vi "practiceImageAnalysis - HH.vi"() -> ()   [LabVIEW 2016]
uses:
  <vilib>/vision/Image Controls.llb/IMAQ Image.ctl
  <vilib>/vision/Measure.llb/Edge Options.ctl
  <vilib>/vision/Measure.llb/Edge Polarity.ctl
  <vilib>/vision/NI_Vision_Development_Module.lvlib
  <vilib>/Analysis/NI_AALPro.lvlib
  <vilib>/Utility/file.llb/Write Delimited Spreadsheet (DBL).vi
panel:
  out "Fitted edge residue":dbl
  out "Fitted edge error":i32
  out "Fitted edge intercept":dbl
  out "Fitted edge slope":dbl
  in  "Linear fit parameter bounds":T1={"slope min"=-inf, "slope max"=inf, "intercept min"=-inf, "intercept max"=inf}
  out "x^2 fit error":i32
  out "Polynomial Coefficients":dbl[](array[numeric])
  out "Residuals":dbl[](array[numeric])
  out "Fitted SD( dI/dR )":dbl[](array[numeric])
  out "Fitted edge locations":dbl[](array[numeric])
  out "residue":dbl
  out "Fit residue vs Z":T2(graph)
  out "Fitted SD dI/dR vs Z":T3(graph)
  out "Fitted radii vs Z":T3(graph)
  out "Processing Image #":i32
  out "Derivative: Normalized Intensity vs Radius":T3(graph)
  out "Selected subarray":T4(plugin-control)
  out "Normalized Intensity vs Radius":cluster{dbl[], dbl[]}(graph)
  in  "nBins":dbl=300.0
  in  "Min":dbl
  in  "Max":dbl=300.0
  out "Fitted Circle":T5 {"Average SNR (dB)" format="%.2f"; "Average Strength" format="%.2f"; "Roundness (Real-World)" format="%.2f"; "Radius (Real-World)" format="%.2f"; "Center (Real-World)"."Y" format="%.2f"; "Center (Real-World)"."X" format="%.2f"; "Radius (Pixels)" format="%.2f"; "Center (Pixels)"."Y" format="%.2f"; "Center (Pixels)"."X" format="%.2f"}
  out "Npixel@Intensity Histogram":T6(graph)
  out "Npixel@phi Histogram":T6(graph)
  out "Npixel@R Histogram":T6(graph)
  in  "Circle ROI Descriptor":T7={"Global Rectangle"=[675, 567, 1751, 1642], "Contours"=[{"ID"=enum."External", "Type"=7, "Coordinates"=[1212, 1104, 85, 537, 0, 0]}]} {"Contours"."Type" items=["No Selection", "Point", "Line", "Rectangle", "Oval", "Polygon", "Freehand Region", "Annulus", "Unused2", "Unused3", "Broken Line", "Freehand Line", "Rotated Rectangle"]}
  in  "Circle Fit Options":T8={"Process"=enum."Get Best Edge", "Step Size"=3.0, "Max Pixel Radius"=3}
  in  "Circle Finding Options":T11={"Search  Direction"=1, "Edge Options"={"Edge Polarity"=2, "Kernel Size"=3, "Width"=3, "Minimum Edge Strength"=10.0, "Interpolation Type"=enum."Bilinear Fixed", "Data Processing Method"=enum."Average"}, "Show Search Area"=FALSE, "Show Search Lines"=FALSE, "Show Edges Found"=FALSE, "Show Result"=TRUE, "Search Area Color"=65280, "Search Lines Color"=255, "Edge Locations Color"=16776960, "Result Color"=65511, "Overlay Group Name"=""} {"Search  Direction" items=["Outside to Inside", "Inside to Outside"]; "Edge Options"."Edge Polarity" items=["All Edges", "Rising Edges", "Falling Edges"]; "Edge Options"."Minimum Edge Strength" format="%.2f"; "Edge Options"."Width" step=2; "Edge Options"."Kernel Size" step=2}
  in  "Pattern Match Settings":T12={"Algorithm"=2, "Number of Matches Requested"=1, "Minimum Match Score"=800.0, "SubPixel Accuracy"=TRUE, "Rotation Angle Ranges"=[], "Show Search Area"=FALSE, "Show Result"=TRUE} {"Rotation Angle Ranges"."End" format="%.1f"; "Rotation Angle Ranges"."Start" format="%.1f"; "Minimum Match Score" min=0 max=1000 format="%.2f"; "Number of Matches Requested" min=1; "Algorithm" items=["All", "Low Discrepancy Sampling", "Grayscale Value Pyramid", "Gradients Pyramid"]}
  out "Template Image":T4
  in  "Coordinate file for image capture":path=path "C:/Users/sciollalab/Desktop/dotCoordinates-captured.csv"
  out "Review":bool
  out "Search running?":bool
  in  "Stop and delete":bool
  out "Images Array":T4[](array[plugin-control])=["image_442_-22_00"]
  in  "error in":errorcluster
  out "error out":errorcluster
  out "Filenames Array":string[](array[string])
  in  "Naming Convention":string="image_442_-22_00.png"
  in  "Images Directory":path=path "C:/Users/sciollalab/Desktop/dots1-12-16-2016/dots_-146,-22"
  # "add linear fit to R vs Z"
  # "fit to a parabola"
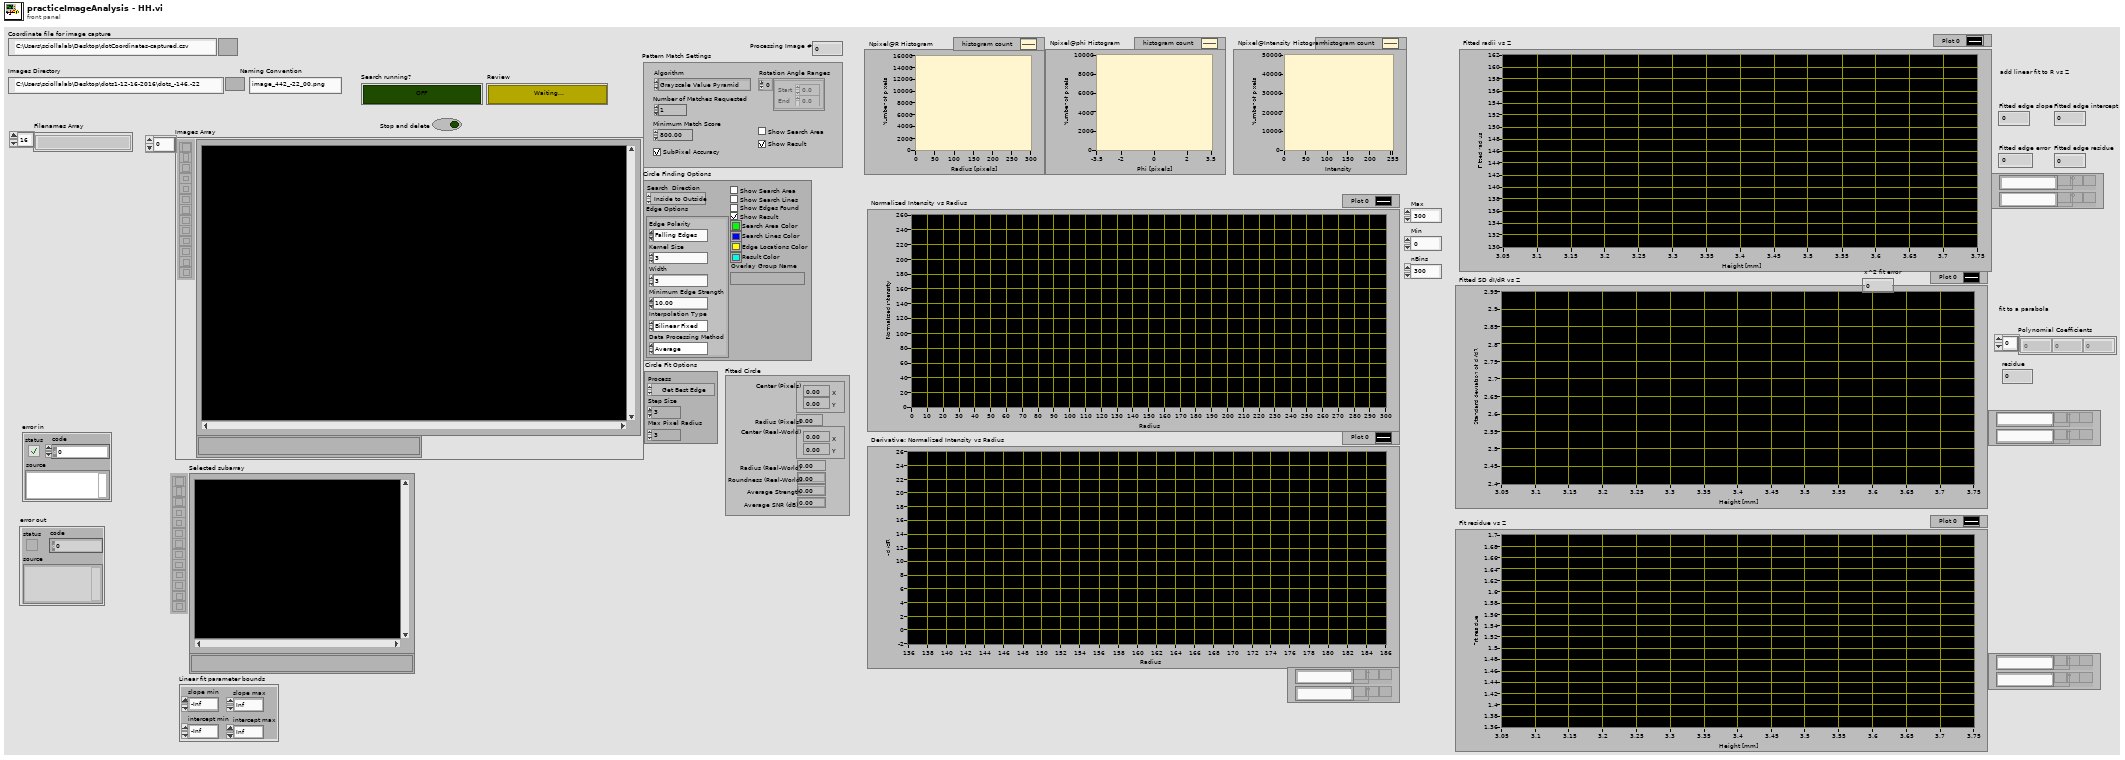
[diagram p1: front panel]
types:
  T1 = cluster{"slope min":dbl, "slope max":dbl, "intercept min":dbl, "intercept max":dbl}
  T2 = cluster{"Image coordinates in lab frame":dbl[], dbl[]}
  T3 = cluster{"Radius bins":dbl[], "Best Gaussian Fit":dbl[]}[]
  T4 = typedef "IMAQ Image.ctl" = refnum<image>
  T5 = cluster{"Center (Pixels)":cluster{"X":sgl, "Y":sgl}, "Radius (Pixels)":dbl, "Center (Real-World)":cluster{"X":sgl, "Y":sgl}, "Radius (Real-World)":dbl, "Roundness (Real-World)":dbl, "Average Strength":dbl, "Average SNR (dB)":dbl}
  T6 = cluster{"X Values":dbl[], "Histogram: h(x)":i32[]}
  T7 = cluster{"Global Rectangle":i32[], "Contours":cluster{"ID":enum32{"External", "Internal"}, "Type":u32, "Coordinates":i32[]}[]}
  T8 = cluster{"Process":enum16{"Get First Edge", "Get First + Last Edge", "Get All Edges", "Get Best Edge"}, "Step Size":dbl, "Max Pixel Radius":i32}
  T9 = typedef "Edge Options.ctl" = cluster{"Edge Polarity":T10, "Kernel Size":u32, "Width":u32, "Minimum Edge Strength":sgl, "Interpolation Type":enum32{"Zero Order", "Bilinear", "Quadratic", "Cubic", "Bilinear Fixed"}, "Data Processing Method":enum32{"Average", "Median"}}
  T10 = typedef "Edge Polarity.ctl" = u32
  T11 = cluster{"Search  Direction":u32, "Edge Options":T9, "Show Search Area":bool, "Show Search Lines":bool, "Show Edges Found":bool, "Show Result":bool, "Search Area Color":u32, "Search Lines Color":u32, "Edge Locations Color":u32, "Result Color":u32, "Overlay Group Name":string}
  T12 = cluster{"Algorithm":i32, "Number of Matches Requested":i32, "Minimum Match Score":sgl, "SubPixel Accuracy":bool, "Rotation Angle Ranges":cluster{"Start":sgl, "End":sgl}[], "Show Search Area":bool, "Show Result":bool}
  T13 = enum16{"cm", "mm", "pixels [mm/pix]", "pixels [um/pix]"}
  T14 = cluster{"Position":cluster{"x":sgl, "y":sgl}, "Angle":sgl, "Scale":sgl, "Score":sgl, "Bounding Box":cluster{"x":sgl, "y":sgl}[]}[]
  T15 = cluster{"Global Rectangle":i32[], cluster{"ID":enum32{"External", "Internal"}, "Type":u32, "Coordinates":i32[]}[]}
  T16 = cluster{"initial amplitude":dbl, "initial center":dbl, "initial standard deviation":dbl, "offset":dbl}
  T17 = cluster{"Image coordinates in lab frame":dbl[], "Residuals":dbl[]}
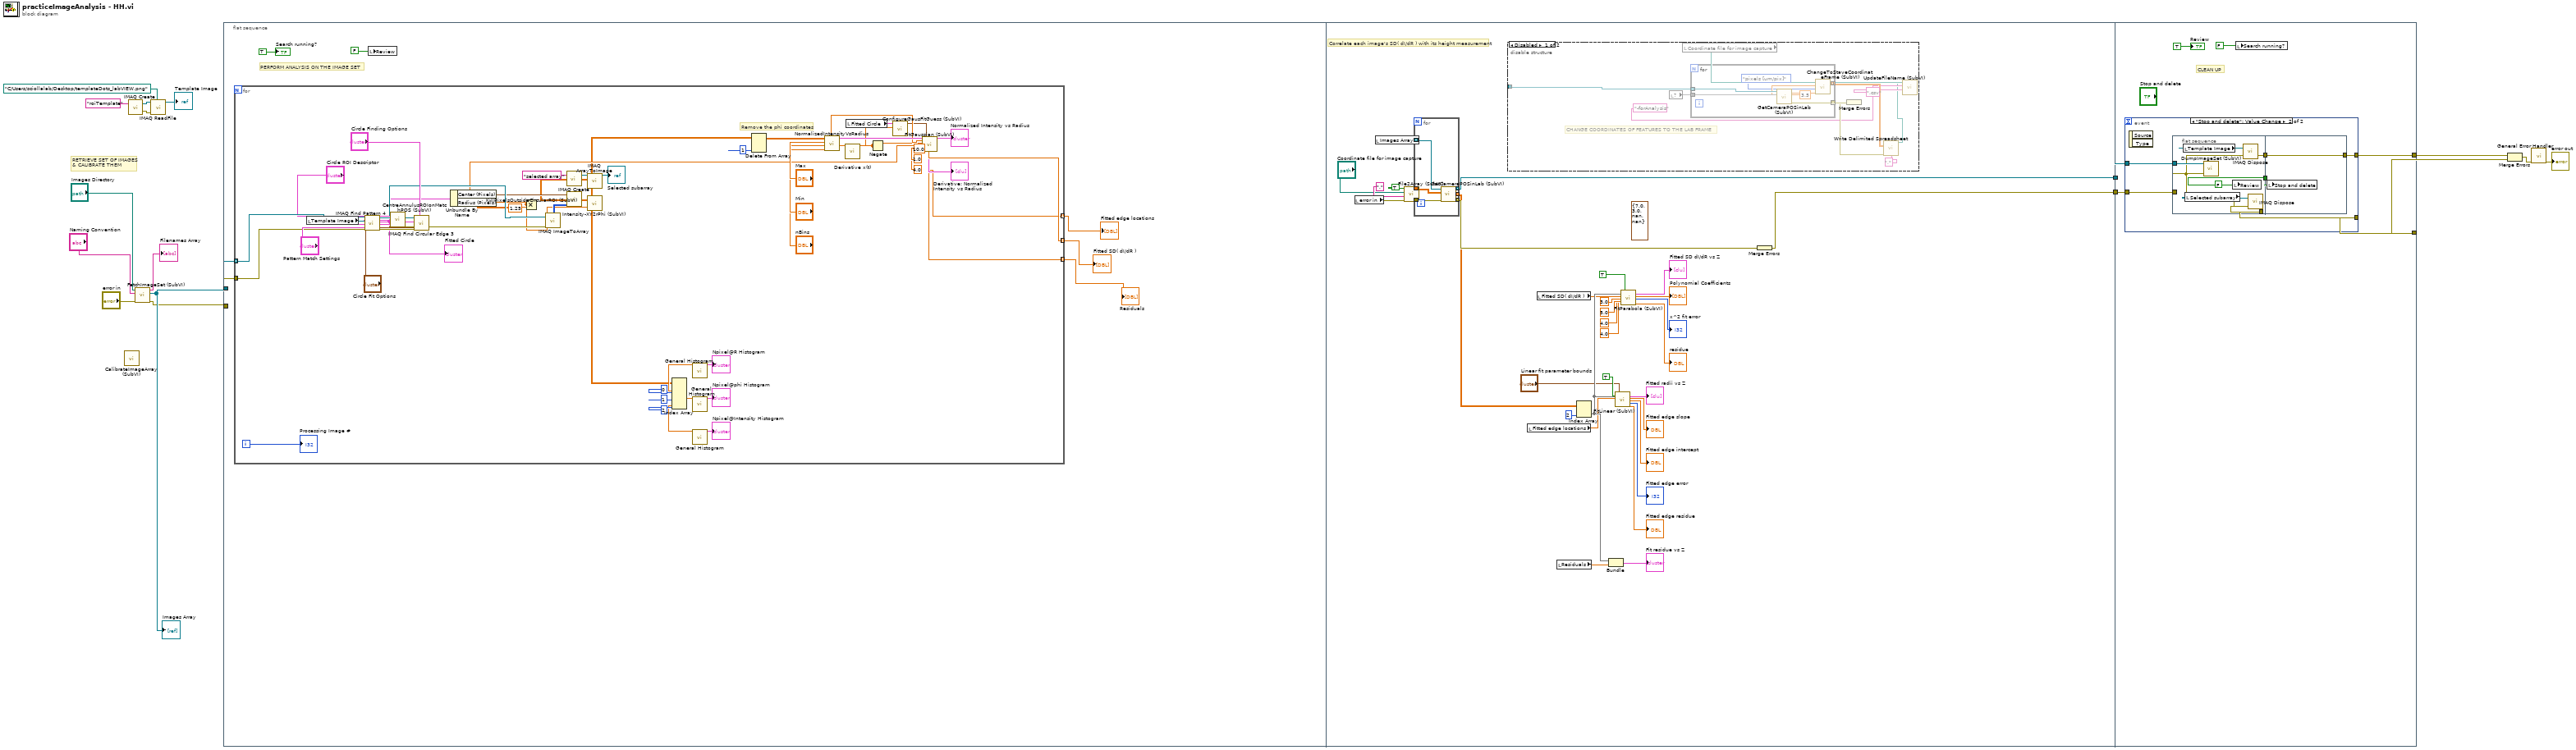
[diagram p0: block diagram]
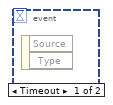
[diagram p3: hidden frame]
diagram:
  # "RETRIEVE SET OF IMAGES\n& CALIBRATE THEM"
  n1 = call "CalibrateImageArray (SubVI).vi"() -> ()  [unwired: 9 in, 2 out]
  n2 = call "IMAQ Create"("Image Name"="roiTemplate") -> ("New Image"=w7:T4, "error out"=w8:errorcluster)  [unwired: 4 in]
  n3 = call "FetchImageSet (SubVI).vi"("error in (no error)"="error in", "Naming Convention"="Naming Convention", "Images Directory"="Images Directory") -> ("error out"=w4:errorcluster, "Image Array"=w10:T4[], "Filenames Array"=→"Filenames Array":string[])  [unwired: 6 in]
  "Images Array" <- w10
  n4 = call "IMAQ ReadFile"("File Path"=path "C:/Users/sciollalab/Desktop/templateDots_labVIEW.png" ("Template File Path"), "error in (no error)"=w8, "Image"=w7) -> ("Image Out"=→"Template Image":T4)  [unwired: 4 in, 4 out]
  n5 = flat-sequence {
    tunnel: w10 -> [w22]
    tunnel: w4 -> [w21]
    tunnel: [w104] -> w3
    tunnel: [w102] -> w2
    tunnel: [w138] -> w12
    tunnel: w3 -> [w137]
    tunnel: w2 -> [w136]
    tunnel: [w135] -> w1
    frame #0 {
      # "PERFORM ANALYSIS ON THE IMAGE SET"
      n6 = for {
        tunnel: w22 -> [w77] mode=indexing
        tunnel: w21 -> [w75]
        tunnel: [w36] -> w19 mode=indexing
        tunnel: [w34] -> w18 mode=indexing
        tunnel: [w33] -> w20 mode=indexing
        i -> [w37]
        # "Remove the phi coordinates"
        n7 = local read "Template Image"() -> (w78:T4)
        n8 = call "IMAQ Find Pattern 4"("Image"=w77, "Template"=w78, "error in"=w75, "Settings"="Pattern Match Settings") -> ("Image Out"=w69:T4, "Matches (pixel)"=w71:T14, "error out"=w68:errorcluster)  [unwired: 5 in, 4 out]
        n9 = call "CentreAnnulusROIonMatchPOS (SubVI).vi"("Matches (pixel)"=w71, "Annulus ROI Descriptor"="Circle ROI Descriptor") -> ("Annulus ROI Descriptor centred on match position"=w70:T15)
        n10 = call "IMAQ Find Circular Edge 3"("Circle Fit Options"="Circle Fit Options", "Options"="Circle Finding Options", "error in (no error)"=w68, "ROI Descriptor"=w70, "Image"=w69) -> ("error out"=w67:errorcluster, "Fitted Circle"=w30:T5, "Image Out"=w59:T4)  [unwired: 2 in, 2 out]
        "Fitted Circle" <- w30
        n11 = Unbundle By Name(w30) -> ("Center (Pixels)"=w56:cluster{"X":sgl, "Y":sgl}, "Radius (Pixels)"=w38:dbl)
        n12 = Multiply(x=w38, y=1.25) -> (x*y=w44:dbl)
        n13 = call "IMAQ ImageToArray"("error in (no error)"=w67, "Image"=w59) -> ("Image Pixels (U8)"=w57:u8[][])  [unwired: 2 in, 4 out]
        n14 = call "IMAQ Create"("Image Name"="selected array") -> ("New Image"=w47:T4)  [unwired: 4 in, 1 out]
        n15 = call "KillPixelsOutsideCircularROI (SubVI).vi"("XY Array"=w57, "Radius*ScaleFactor"=w44, "Center (Pixels)"=w56) -> ("subarray"=w46:dbl[][])
        n16 = call "IMAQ ArrayToImage"("Image Pixels (U8)"=w46, "Image"=w47) -> ("Image Out"=→"Selected subarray":T4)  [unwired: 8 in, 1 out]
        n17 = call "Intensity-XY2rPhi (SubVI).vi"("Radius*Scale Factor"=w44, "XY Array"=w46) -> ("2D Array: r, phi, intensity"=w32:dbl[][])  [unwired: 1 out]
        n18 = Index Array(array=w32, index (col) #1=0 ("disabled index (col)"), index (col) #2=1 ("index (col)"), index (col) #3=2 ("index (col)")) -> (element #1=w55:dbl[], element #2=w60:dbl[], element #3=w54:dbl[])  [unwired: 3 in]
        n19 = call <vilib>:"General Histogram.vi"("X"=w55) -> ("Histogram Graph"=→"Npixel@R Histogram":T6)  [unwired: 10 in, 4 out]
        n20 = call <vilib>:"General Histogram.vi"("X"=w60) -> ("Histogram Graph"=→"Npixel@phi Histogram":T6)  [unwired: 10 in, 4 out]
        n21 = call <vilib>:"General Histogram.vi"("X"=w54) -> ("Histogram Graph"=→"Npixel@Intensity Histogram":T6)  [unwired: 10 in, 4 out]
        n22 = Delete From Array(array=w32, index (col)=1 ("disabled index (col)")) -> (array with subset deleted=w52:dbl[][])  [unwired: 2 in, 1 out]
        n23 = call "NormalizedIntensityVsRadius.vi"("nBins"="nBins", "Min"="Min", "Max"="Max", "Input Array (r,I)"=w52) -> ("Normalized Intensity"=w42:dbl[], "Radius bins"=w40:dbl[], "Normalized Intensity vs Radius"=w43:cluster{dbl[], dbl[]})  [unwired: 5 in]
        n24 = call <vilib>:"Derivative x(t).vi"("X"=w42) -> ("dX/dt"=w41:dbl[])  [unwired: 9 in, 1 out]
        n25 = local read "Fitted Circle"() -> (w29:T5)
        n26 = Negate(x=w41) -> (-x=w28:dbl[])
        n27 = call "ConfigureGausFitGuess (SubVI).vi"("Array"=w28, "Fitted Circle"=w29) -> ("initial guess out"=w31:T16)  [unwired: 9 in]
        n28 = call "FitGaussian (SubVI).vi"("Normalized Intensity vs Radius in"=w43, "x values"=w40, "y values"=w28, "Estimated mean"=w38, "Estimated width"=10.0, "initial guess"=w31, "Nsigma Low"=1.0, "Nsigma High"=4.0) -> ("data plot"=→"Normalized Intensity vs Radius":cluster{dbl[], dbl[]}, "derivative data plot with Gaussian fit"=→"Derivative: Normalized Intensity vs Radius":T3, "center"=w33:dbl, "standard deviation"=w36:dbl, "residue"=w34:dbl)  [unwired: 6 in, 1 out]
        "Processing Image #" <- w37
      }
      "Fitted edge locations" <- w20
      "Fitted SD( dI/dR )" <- w19
      "Residuals" <- w18
      n29 = local write "Review"(FALSE ("Review")) -> ()
      "Search running?" <- TRUE ("Search running?")
    }
    frame #1 {
      (unwired) T16 {"initial amplitude"=7.0, "initial center"=3.0, "initial standard deviation"=nan, "offset"=nan} ("initial guess")
      # "Correlate each image's SD( dI/dR ) with its height measurement"
      n30 = local read "error in"() -> (w111:errorcluster)
      n31 = local read "Images Array"() -> (w107:T4[])
      n32 = call "File2Array (SubVI).vi"("error in (no error) in"=w111, "File delimiter"=",", "Source array file"="Coordinate file for image capture", "Load array from file?"=TRUE) -> ("error in (no error) out"=w105:errorcluster, "Loaded array"=w106:dbl[][])  [unwired: 6 in]
      n33 = for {
        tunnel: w107 -> [w117] mode=indexing
        tunnel: w106 -> [w116]
        tunnel: w105 -> [w115]
        tunnel: [w114] -> w104 mode=indexing
        tunnel: [w113] -> w103 mode=indexing
        tunnel: [w112] -> w91 mode=indexing
        n34 = call "GetCameraPOSinLab (SubVI).vi"("error in (no error)"=w115, "Loaded array"=w116, "Refnum in"=w117) -> ("error out"=w113:errorcluster, "Image coordinates in lab frame"=w112:dbl[], "Refnum out"=w114:T4)  [unwired: 6 in]
      }
      n35 = disable-structure shown="Disabled" {
        disable-tunnel: _ -> [w119 _]
        frame Disabled {
          # "CHANGE COORDINATES OF FEATURES TO THE LAB FRAME"
          n36 = local read item#-1() -> (w127)
          n37 = local read "Coordinate file for image capture"() -> (w122:path)
          n38 = for {
            tunnel: w119 -> [w134] mode=indexing
            tunnel: w127 -> [w133]
            tunnel: [w129] -> w124 mode=concatenating
            tunnel: [w128] -> w126 mode=indexing
            n39 = call "GetCameraPOSinLab (SubVI).vi"("Loaded array"=w133, "Refnum in"=w134) -> ("error out"=w128:errorcluster, "Image coordinates in lab frame"=w132:dbl[])  [unwired: 7 in, 1 out]
            n40 = call "ChangeToStaveCoordinateFrame (SubVI).vi"("Image Origin in XYZ Stage Coords [mm]"=w132, "Units"=T13."pixels [um/pix]", "Pixel resolution"=3.5) -> ("Array (stage frame, mm)"=w129:dbl[][])  [unwired: 3 in]
          }
          n41 = Merge Errors(w126) -> (w123:errorcluster)
          n42 = call "UpdateFileName (SubVI).vi"("File Extension"=".csv" ("regular expression"), "Append to Filename"="-forAnalysis" ("name or relative path"), "Path and filename"=w122) -> ("Updated Path"=w118:path)  [unwired: 8 in]
          n43 = call-poly <vilib>:"Write Delimited Spreadsheet.vi"("file path (dialog if empty)"=w118, "2D data"=w124, "error in (no error)"=w123, "delimiter (\\t)"="," ("delimiter (\\t)")) -> ()  [unwired: 10 in, 2 out]
        }
        frame Enabled {
        }
      }
      n44 = local read "Fitted edge locations"() -> (w87:dbl[])
      n45 = local read "Fitted SD( dI/dR )"() -> (w79:dbl[])
      n46 = local read "Residuals"() -> (w94:dbl[])
      n47 = Index Array(array=w91, index (col)=2 ("disabled index (col)")) -> (element=w88:dbl[])  [unwired: 1 in]
      n48 = Bundle("Image coordinates in lab frame"=w88, "Residuals"=w94) -> (→"Fit residue vs Z":T17)  [unwired: 1 in]
      n49 = call "FitLinear (SubVI).vi"("x values"=w88, "y values"=w87, "parameter bounds"="Linear fit parameter bounds", "Use all points"=TRUE) -> ("derivative data plot with linear fit"=→"Fitted radii vs Z":T3, "slope"=→"Fitted edge slope":dbl, "intercept"=→"Fitted edge intercept":dbl, "error"=→"Fitted edge error":i32, "residue"=→"Fitted edge residue":dbl)  [unwired: 10 in, 1 out]
      n50 = call "FitParabola (SubVI).vi"("x values"=w88, "y values"=w79, "Estimated mean"=3.0 ("Radius"), "Estimated width"=5.0, "Nsigma Low"=4.0, "Use all points"=TRUE, "Nsigma High"=4.0) -> ("derivative data plot with Gaussian fit"=→"Fitted SD dI/dR vs Z":T3, "Polynomial Coefficients"=→"Polynomial Coefficients":dbl[], "error"=→"x^2 fit error":i32, "residue"=→"residue":dbl)  [unwired: 8 in, 1 out]
      n51 = Merge Errors(w103) -> (w102:errorcluster)
    }
    frame #2 {
      # "CLEAN UP"
      n52 = event shown="[1] \"Stop and delete\": Value Change" {
        selector: _ -> [_ _]
        dyn-events: _ -> [_ _]
        timeout: _ -> [_ _]
        tunnel: [_ w146] -> w138
        tunnel: w137 -> [_ w143]
        tunnel: w136 -> [_ w142]
        tunnel: [_ w141] -> w135
        event Timeout {
          n53 = event-data() -> ()  [unwired: 1 in, 2 out]
        }
        event "Stop and delete": Value Change {
          n54 = event-data() -> ()  [unwired: 1 in, 2 out]
          n55 = flat-sequence {
            tunnel: [w153] -> w145
            tunnel: [w152] -> w144
            tunnel: w143 -> [w151]
            tunnel: w142 -> [w149]
            tunnel: [w147] -> w141
            tunnel: [w156] -> w146
            tunnel: w145 -> [w156]
            tunnel: w144 -> [w155]
            frame #0 {
              w152 = FALSE ("Review")
              n56 = local read "Template Image"() -> (w154:T4)
              n57 = local read "Selected subarray"() -> (w150:T4)
              n58 = call "DumpImageSet (SubVI).vi"("error in (no error)"=w149, "Calibrated Image Array"=w151) -> ("error out"=w148:errorcluster)  [unwired: 6 in]
              n59 = local write "Review"(w152) -> ()
              n60 = call "IMAQ Dispose"("Image"=w154, "error in (no error)"=w148) -> ("error out"=w153:errorcluster)  [unwired: 4 in]
              n61 = call "IMAQ Dispose"("Image"=w150, "error in (no error)"=w148) -> ("error out"=w147:errorcluster)  [unwired: 4 in]
            }
            frame #1 {
              n62 = local write "Stop and delete"(w155) -> ()
            }
          }
        }
      }
      n63 = local write "Search running?"(FALSE ("Search running?")) -> ()
      "Review" <- TRUE ("Review")
    }
  }
  n64 = Merge Errors(w12, w1) -> (w11:errorcluster)
  n65 = call <vilib>:"General Error Handler.vi"("error in (no error)"=w11) -> ("error out"=→"error out":errorcluster)  [unwired: 10 in, 4 out]
